vi "Array Limit.vi"(9 "index":i32, 11 "array":string[](array[string])) -> (2 "x = y?":bool)   [LabVIEW 2014, in "Master.lvclass"]
uses:
  Master/Master.lvclass
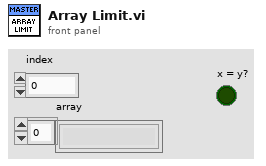
[diagram p1: front panel]
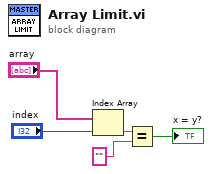
[diagram p0: block diagram]
diagram:
  n1 = Index Array(array="array", index="index") -> (element=w3:string)
  n2 = Equal?(x=w3, y="") -> (x = y?=→"x = y?":bool)
